vi "CreateHTML.vi"(0 "reference in":refnum<class "Numeric.lvclass">, 2 "VI Name":string, 5 "error in (no error)":errorcluster) -> (13 "script dependencies":string[](array[string]), 14 "reference out":refnum<class "Numeric.lvclass">, 15 "HTML":string, 16 "js variables":string, 17 "js code for controls":string, 18 "js code for indicators":string, 19 "error out":errorcluster)   [LabVIEW 2014, in "Numeric.lvclass"]
uses:
  Numeric.lvclass
  Object_class/Object.lvclass
  Control_class/Control.lvclass
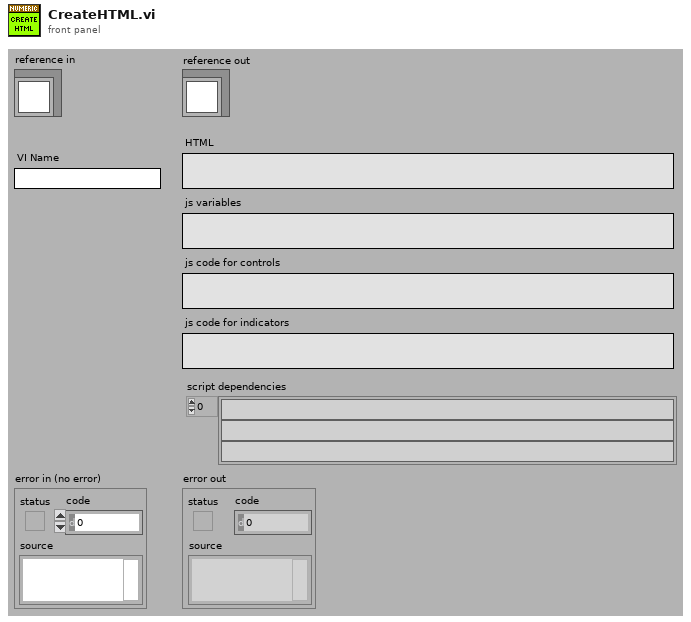
[diagram p1: front panel]
types:
  T1 = typedef "Object.lvclass/Attributes.ctl" = cluster{"UID":i32, "Type":string, "Coordinates":T2}
  T2 = typedef "Object.lvclass/Coordinates.ctl" = cluster{"Left":i32, "Top":i32, "Height":u32, "Width":u32}
  T3 = typedef "Control.lvclass/Attributes.ctl" = cluster{"Description":string, "Indicator":bool, "Default Value":variant, "Control Index":i32, "Label":refnum<class "Text.lvclass">, "Caption":refnum<class "Text.lvclass">, "Use Picture":bool, "Image 1":T4, "Image 2":T4}
  T4 = typedef "imagedata.ctl" = cluster{"image type":i32, "image depth":i32, "image":u8[], "mask":u8[], "colors":u32[], "Rectangle":cluster{"left":i16, "top":i16, "right":i16, "bottom":i16}}
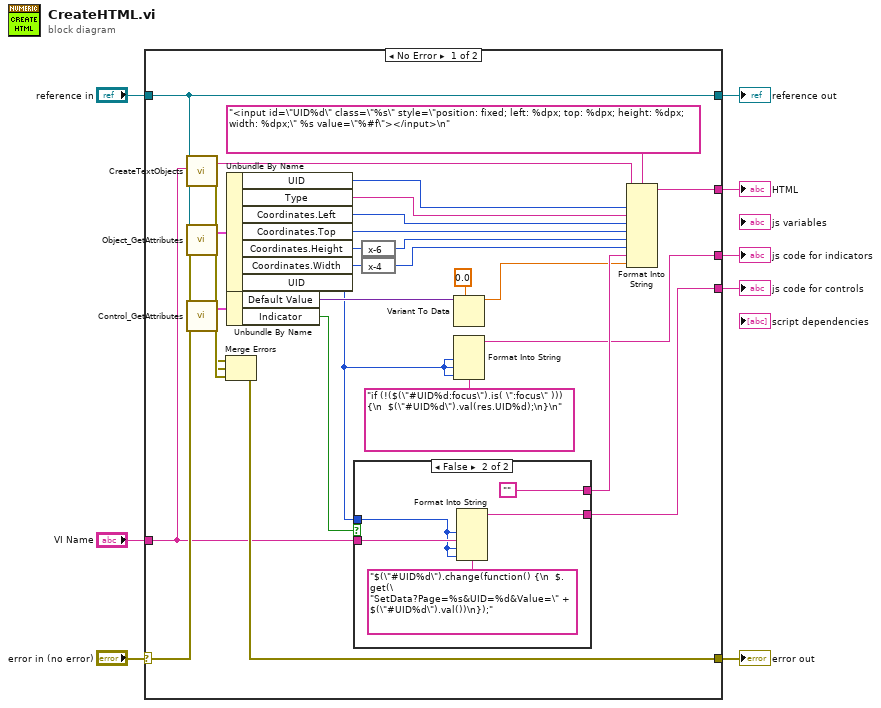
[diagram p0: block diagram]
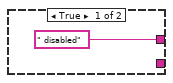
[diagram p2: hidden frame]
diagram:
  n1 = case shown="No Error" "error in (no error)" {
    selector: "error in (no error)" -> [w37 w45]
    tunnel: [w33 w45] -> w7
    tunnel: [w10 w44] -> w5
    tunnel: "reference in" -> [w10 w44]
    tunnel: [w27 _] -> w4
    tunnel: [w13 _] -> w3
    tunnel: [w18 _] -> w2
    tunnel: "VI Name" -> [w9 _]
    frame No Error {
      n2 = call-dynamic "CreateTextObjects.vi"("reference in"=w10, "VI Name"=w9) -> ("HTML"=w11:string, "error out"=w34:errorcluster)  [unwired: 15 in, 1 out]
      n3 = call "Object_GetAttributes.vi"("reference in"=w10, "error in (no error)"=w37) -> ("Data"=w26:T1, "error out"=w35:errorcluster)  [unwired: 14 in, 2 out]
      n4 = call "Control_GetAttributes.vi"("reference in"=w10, "error in (no error)"=w37) -> ("Data"=w21:T3, "error out"=w36:errorcluster)  [unwired: 14 in, 2 out]
      n5 = Merge Errors(w34, w35, w36) -> (w33:errorcluster)
      n6 = Unbundle By Name(w26) -> ("UID"=w31:i32, "Type"=w30:string, "Coordinates.Left"=w29:i32, "Coordinates.Top"=w28:i32, "Coordinates.Height"=w25:u32, "Coordinates.Width"=w23:u32, "UID"=w12:i32)
      n7 = Unbundle By Name(w21) -> ("Default Value"=w16:variant, "Indicator"=w20:bool)
      n8 = case shown="False" w20 {
        tunnel: [" disabled" ""] -> w19
        tunnel: w12 -> [_ w40]
        tunnel: w9 -> [_ w43]
        tunnel: [_ w39] -> w18
        frame True {
        }
        frame False {
          n9 = Format Into String(format string="$(\"#UID%d\").change(function() {\n  $.get(\"SetData?Page=%s&UID=%d&Value=\" + $(\"#UID%d\").val())\n});", w40, w43, w40, w40) -> (resulting string=w39:string)  [unwired: 2 in, 1 out]
        }
      }
      n10 = expression code="x-6"(w25) -> (w24:u32)
      n11 = expression code="x-4"(w23) -> (w22:u32)
      n12 = Variant To Data(type=0.0, Variant=w16) -> (data=w15:dbl)  [unwired: 1 in, 1 out]
      n13 = Format Into String(format string="if (!($(\"#UID%d:focus\").is( \":focus\" ))) {\n  $(\"#UID%d\").val(res.UID%d);\n}\n", w12, w12, w12) -> (resulting string=w13:string)  [unwired: 2 in, 1 out]
      n14 = Format Into String(format string="<input id=\"UID%d\" class=\"%s\" style=\"position: fixed; left: %dpx; top: %dpx; height: %dpx; width: %dpx;\" %s value=\"%#f\"></input>\n", initial string=w11, w31, w30, w29, w28, w24, w22, w19, w15) -> (resulting string=w27:string)  [unwired: 1 in, 1 out]
    }
    frame Error {
    }
  }
  "error out" <- w7
  "reference out" <- w5
  "HTML" <- w4
  "js code for controls" <- w2
  "js code for indicators" <- w3
